vi "Orbit and Timebase Plot (Simulated)_KSS.vi"(8 "error in":errorcluster) -> (0 "error out":errorcluster, 3 "XY Graph":cluster{"probe x":dbl[], "probe y":dbl[]}[](graph))   [LabVIEW 2020]
doc: "This VI demonstrates how to display orbit and timebase plots with a simulated signal.\n\n<B>INSTRUCTIONS</B>:\n1. Specify the <B>sampling info</B>, <B>signal rotating speed</B> and <B>order components</B> contained in the x- and y-axis signals.\n2. For filtered plot, you can specify the <B>orders to display</B> and <B>bandwidth [order]</B>. \n3. Specify the shaft rotating direction, probe orientation and channel pair information in <B> channel properties</B>.\n4. Specify when the display starts and ends to update by setting <B>start [rev]</B> and <B>end [rev]</B> in <B>segment settings</B>.\n5. Specify the <B>timebase buffer size (rev)</B> and <B>orbit buffer size (rev)</B> if you want to view more revolution signals on the plot.\n6. Run the VI.\n\n<B>VIs USED IN THIS EXAMPLE</B>:\n1. OAT Analog Tacho Process.vi\n2. OAT Convert to Even Angle Signal.vi\n3. OAT Order Magnitude and Phase.vi\n4. OAT AC DC Separation.vi\n5. SVX Orbit and Timebase Plot.vi\n6. SVX Combine Filtered and Unfiltered Plots.vi\n7. SVX Buffer Orbit Timebase Plot.vi"
uses:
  <vilib>/addons/_NISVFA/_Shared subVIs/Controls/svc_Channel Info.ctl
  <vilib>/addons/_NISVFA/_Shared subVIs/Controls/svc_Engineering Units Text Ring.ctl
  <vilib>/addons/_NISVFA/_Shared subVIs/Controls/svc_Weighting Filter Text Ring.ctl
  <vilib>/addons/_XControls/Timebase Plot/SVX Timebase.xctl
  <vilib>/addons/_XControls/Orbit Plot/SVX Orbit.xctl
  <vilib>/addons/Sound and Vibration/Order Analysis/Data Presentation/SubVIs/OAT MCM Channel Property.ctl
  <vilib>/addons/_NISVFA/_Shared subVIs/Controls/svc_Window [Dual FFT].ctl
  <vilib>/addons/Sound and Vibration/svt_Calibration/SVL Scale Voltage to EU (N Ch - 1 Info).vi
  <vilib>/addons/Sound and Vibration/svt_Calibration/SVL Scale Voltage to EU (1 Ch).vi
  <vilib>/addons/_NISVFA/_Shared subVIs/Common/svc_Set SV Channel Info.vi
  <vilib>/addons/_NISVFA/_Shared subVIs/Common/svc_Set SV Channel Info (variant).vi
  <vilib>/addons/_NISVFA/_Shared subVIs/Common/SVL Set dB Reference (variant).vi
  <vilib>/addons/_NISVFA/_Shared subVIs/Common/svc_Engineering Units to Unit Label.vi
  <vilib>/addons/_NISVFA/_Shared subVIs/Common/svc_Compute Scale Factor to Convert V to EU.vi
  <vilib>/addons/_NISVFA/_Shared subVIs/Common/svc_Compute Scale Factor to Convert C to EU.vi
  <vilib>/addons/_NISVFA/_Shared subVIs/Common/svc_Set dB ref if Pascal.vi
  <vilib>/addons/_NISVFA/_Shared subVIs/Common/svc_Caller VI Returned in Error Source.vi
  <vilib>/addons/Sound and Vibration/Order Analysis/Tach Process/OAT Analog Tacho Process (1 Tacho).vi
  <vilib>/addons/Sound and Vibration/Order Analysis/Resample Order Tracking/OAT Convert to Even Angle Signal (N Channels).vi
  <vilib>/addons/Sound and Vibration/Order Analysis/Utility/OAT AC DC Separation (N Channels).vi
  <vilib>/addons/Sound and Vibration/Order Analysis/Data Presentation/SVX Orbit and Timebase Plot (Unfiltered).vi
  <vilib>/addons/Sound and Vibration/Order Analysis/Resample Order Tracking/OAT Order Magnitude and Phase (Even Angle Signal, N Channels).vi
  <vilib>/addons/Sound and Vibration/Order Analysis/Data Presentation/SVX Orbit and Timebase Plot (Filtered) (N Ch - M Orders).vi
  <vilib>/addons/Sound and Vibration/Order Analysis/Resample Order Tracking/OAT Full Spectrum (Orbit Plot).vi
  <vilib>/addons/Sound and Vibration/svt_Calibration/SoundVib_Calibration.lvlib
  <vilib>/addons/Sound and Vibration/Order Analysis/Tach Process/SoundVib_TachProcess.lvlib
  <vilib>/addons/Sound and Vibration/Order Analysis/Resample Order Tracking/SoundVib_OrderTracking.lvlib
  <vilib>/addons/Sound and Vibration/Order Analysis/Utility/SoundVib_OAUtility.lvlib
  <vilib>/addons/Sound and Vibration/Order Analysis/Data Presentation/SoundVib_MCMDisplay.lvlib
panel:
  out "orbit/timebase plot out":T1(array[cluster])
  out "subarray":T2(array[cluster])
  in  "channel properties":T3[](array[typedef]) {"probe angle [deg]" max=360; "direction" items=["CCW", "CW"]}
  in  "segment settings":cluster{"start [rev]":dbl, "end [rev]":dbl}={"start [rev]"=0.0, "end [rev]"=inf}
  in  "orbit buffer size (rev)":u32=8
  in  "timebase buffer size (rev)":u32=8
  in  "orders to display":dbl[](array[numeric])=[1.0] format="%.2f"
  in  "y axis order components":T4(array[cluster])=[{"order"=1, "amplitude"=0.5, "phase (deg)"=90.0, "order envelop"=0}, {"order"=2, "amplitude"=1.0, "phase (deg)"=45.0, "order envelop"=2}] {"order envelop" items=["None", "Sine", "Triangle"]}
  in  "channel info":T5={"sensor sensitivity"=1000.0, "engineering units"=1, "dB reference"=1.0, "custom label"="EU", "weighting filter"=0, "pregain"=0.0} {"pregain" format="%.2f"; "weighting filter" items=["Linear", "A-weighting", "B-weighting", "C-weighting", "ITU-R 468-4", "Dolby", "CCITT", "C-message", "Wb", "Wc", "Wd", "We", "Wf", "Wh", "Wj", "Wk", "Wm", "AES17 20 kHz lowpass", "AES17 40 kHz lowpass", "AES17 20 kHz highpass", "AES17 40 kHz highpass"]; "dB reference" format="%^.1e"; "engineering units" items=["custom..."=0, "V"=1, "A"=21, "C"=30, "pC"=31, "s"=32, "-"=29, "Pa"=2, "N"=20, "g"=3, "m/s^2"=4, "m/s"=5, "m"=6, "mm/s"=12, "mm"=13, "micron/s"=14, "micron"=15, "in/s^2"=7, "in/s"=8, "in"=9, "mil/s"=10, "mil"=11, "rad/s^2"=16, "rad/s"=17, "rad"=18, "deg/s^2"=26, "deg/s"=27, "deg"=28, "RPM"=22, "cycle/s^2"=23, "Hz"=24, "cycle"=25, "strain"=19]; "sensor sensitivity" format="%#_5f"}
  in  "x axis order components":T4(array[cluster])=[{"order"=1, "amplitude"=1.0, "phase (deg)"=0.0, "order envelop"=0}, {"order"=2, "amplitude"=0.5, "phase (deg)"=0.0, "order envelop"=2}] {"order envelop" items=["None", "Sine", "Triangle"]}
  in  "sampling info":T8={"sampling frequency"=10000.0, "duration [s]"=10.0} {"sampling frequency" format="%#_6p"}
  in  "signal rotating speed":u16(ring)=3 items=["3000 RPM", "1000-6000 RPM", "6000-1000 RPM", "1000-6000-1000 RPM"]
  in  "bandwidth [order]":dbl=1.0 format="%.2f"
  in  "Tab Control":T9(tab)
  out "Speed profile":cluster{"time [s]":dbl[], "speed [RPM]":dbl[]}(graph)
  out "Vibration signals":waveform(dbl)[](graph)
  out "Timebase Plot":T10(xcontrol)
  out "Orbit Plot":T1(xcontrol)
  out "Full Spectrum":T11(graph)
  # "Simulated Signal Basic Info"
  # "X and Y axes Components\nin Simulated Signal"
  # "Plot Settings"
  # "Filtered Plot Settings"
  # "Channel Settings"
  # "Select Help»Show Context Help and move the cursor over the VI icon for more information."
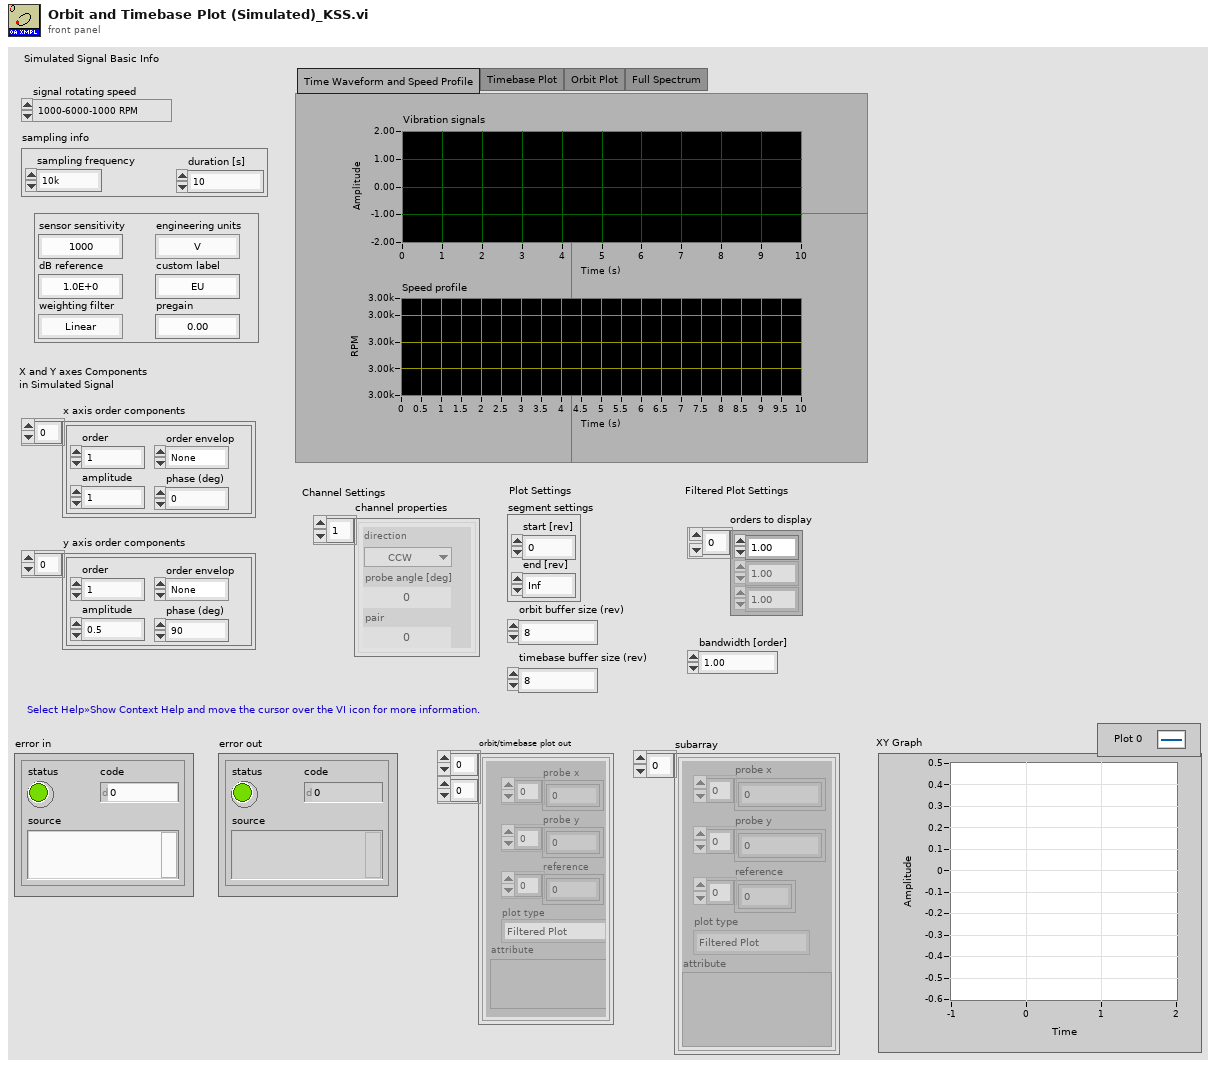
[diagram p1: front panel]
types:
  T1 = cluster{"probe x":dbl[], "probe y":dbl[], "reference":dbl[], "plot type":enum16{"Filtered Plot", "Unfiltered Plot"}, "attribute":variant}[][]
  T2 = cluster{"probe x":dbl[], "probe y":dbl[], "reference":dbl[], "plot type":enum16{"Filtered Plot", "Unfiltered Plot"}, "attribute":variant}[]
  T3 = typedef "OAT MCM Channel Property.ctl" = cluster{"direction":u16, "probe angle [deg]":u16, "pair":u16}
  T4 = cluster{"order":i32, "amplitude":dbl, "phase (deg)":dbl, "order envelop":u16}[]
  T5 = typedef "svc_Channel Info.ctl" = cluster{"sensor sensitivity":dbl, "engineering units":T6, "dB reference":dbl, "custom label":string, "weighting filter":T7, "pregain":dbl}
  T6 = typedef "svc_Engineering Units Text Ring.ctl" = u16
  T7 = typedef "svc_Weighting Filter Text Ring.ctl" = u16
  T8 = cluster{"sampling frequency":dbl, "duration [s]":dbl}
  T9 = enum32{"Time Waveform and Speed Profile", "Timebase Plot", "Orbit Plot", "Full Spectrum"}
  T10 = cluster{"X":dbl[], "Y":dbl[], "reference":dbl[], "plot type":enum16{"Filtered Plot", "Unfiltered Plot"}, "attribute":variant}[][]
  T11 = cluster{"Order 0":dbl, "dOrder":dbl, "magnitude":dbl[]}[]
  T12 = typedef "svc_Window [Dual FFT].ctl" = u32
  T13 = typedef "SoundVib_TachProcess.lvlib/speed profile.ctl" = cluster{"time [s]":dbl[], "speed [RPM]":dbl[]}
  T14 = typedef "svc_Resampled Channel Info.ctl" = cluster{"channel name":string, "description":string, " channel info":T5}
  T15 = typedef "OAT Position Info.ctl" = cluster{"positions [s]":dbl[], "samples/rev":dbl}
  T16 = cluster{"time/rev/rpm":dbl[], "magnitude":dbl[]}[][]
  T17 = typedef "svc_Spectrum Info.ctl" = cluster{"channel name":string, "description":string, "x-axis units":T18, "spectral info":cluster{"spectrum type":T19, "linear/dB":enum16{"linear", "dB"}, "window":u16, "window size":i32, "FFT size":i32}, "engineering units":T6, "custom label":string, "dB reference [EU]":dbl, "peak units":enum16{"rms", "peak", "peak-peak"}, "weighting filter":T7, "spectral density?":bool, "unit label":string, "spectrum skewed?":bool, "complimentary spectrum units":T20}
  T18 = typedef "svc_X-Axis Units.ctl" = u16
  T19 = typedef "svc_Spectrum Type.ctl" = enum16{"FFT Spectrum [complex]", "Amplitude [Magnitude]", "Power [Magnitude^2]", "Cross Spectrum [complex]", "Frequency Response [Complex]"}
  T20 = typedef "svc_Complimentary Spectrum Units.ctl" = enum16{"none", "radians", "degrees", "cycles", "imaginary"}
  T21 = cluster{"forward":cluster{"Order 0":dbl, "dOrder":dbl, "magnitude":dbl[]}, "reverse":cluster{"Order 0":dbl, "dOrder":dbl, "magnitude":dbl[]}}
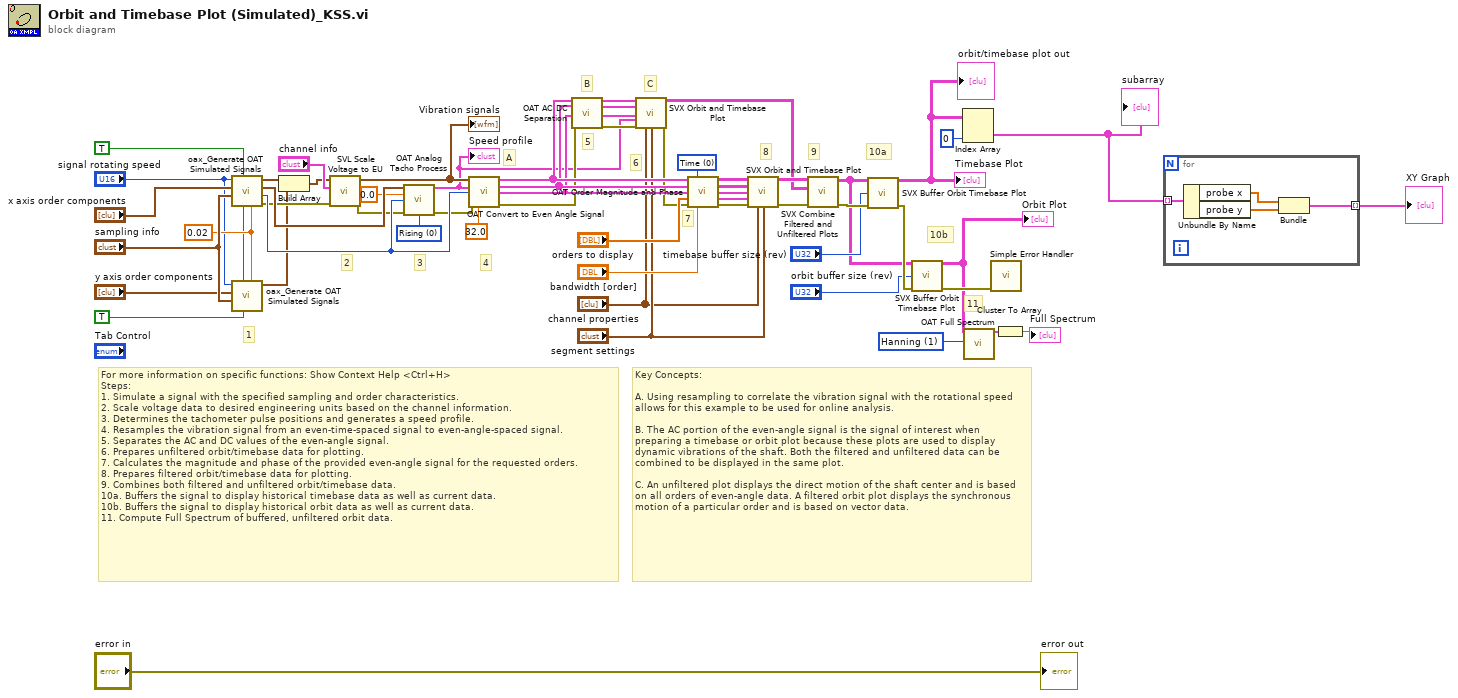
[diagram p0: block diagram]
diagram:
  w9 = T12 1 items=["None"=0, "Hanning"=1, "Hamming"=2, "Blackman-Harris"=3, "Exact Blackman"=4, "Blackman"=5, "Flat Top"=6, "4 Term B-Harris "=7, "7 Term B-Harris"=8, "Low Sidelobe"=9, "Force - Exponential"=10, "Force"=64, "Exponential"=65, "Blackman Nuttall"=11, "Triangle"=30, "Bartlett-Hanning"=31, "Bohman"=32, "Parzen"=33, "Welch"=34, "Kaiser"=60, "Dolph-Chebyshev"=61, "Gaussian"=62] ("window (Hanning)")
  w29 = u16 0 items=["Time", "Revolution", "RPM"] ("X axis selection")
  w39 = u16 0 items=["Rising", "Falling"] ("slope (Rising)")
  w47 = 0.02 ("noise level")
  w46 = TRUE ("add noise?")
  w45 = TRUE ("reset?")
  # "10a"
  # "11"
  # "C"
  # "B"
  # "A"
  # "Key Concepts:\n\nA. Using resampling to correlate the vibration signal with the rotational speed allows for this example to be used for online analysis.\n\nB. The AC portion of the even-angle signal is the signal of interest when preparing a timebase or orbit plot because these plots are used to display dynamic vibrations of the shaft. Both the filtered and unfiltered data can be combined to be displayed in the same plot.\n\nC. An unfiltered plot displays the direct motion of the shaft center and is based on all orders of even-angle data. A filtered orbit plot displays the synchronous motion of a particular order and is based on vector data."
  # "10b"
  # "9"
  # "8"
  # "7"
  # "6"
  # "5"
  # "For more information on specific functions: Show Context Help <Ctrl+H>\nSteps:\n1. Simulate a signal with the specified sampling and order characteristics.\n2. Scale voltage data to desired engineering units based on the channel information.\n3. Determines the tachometer pulse positions and generates a speed profile.\n4. Resamples the vibration signal from an even-time-spaced signal to even-angle-spaced signal.\n5. Separates the AC and DC values of the even-angle signal.\n6. Prepares unfiltered orbit/timebase data for plotting.\n7. Calculates the magnitude and phase of the provided even-angle signal for the requested orders.\n8. Prepares filtered orbit/timebase data for plotting.\n9. Combines both filtered and unfiltered orbit/timebase data.\n10a. Buffers the signal to display historical timebase data as well as current data. \n10b. Buffers the signal to display historical orbit data as well as current data. \n11. Compute Full Spectrum of buffered, unfiltered orbit data."
  # "4"
  # "3"
  # "2"
  # "1"
  n1 = call <vilib>:"oax_Generate OAT Simulated Signals.vi"("noise level"=w47, "add noise?"=w46, "reset?"=w45, "sampling info"="sampling info", "ordercomponents"="x axis order components", "signal rotating speed"="signal rotating speed") -> ("error out"=w51:errorcluster, "pulse/revolution"=w57:i32, "Tach Signal"=w58:waveform(dbl), "Vibration Signal"=w52:waveform(dbl))  [unwired: 2 in]
  n2 = call <vilib>:"oax_Generate OAT Simulated Signals.vi"("noise level"=w47, "add noise?"=w46, "reset?"=w45, "sampling info"="sampling info", "ordercomponents"="y axis order components", "signal rotating speed"="signal rotating speed") -> ("Vibration Signal"=w42:waveform(dbl))  [unwired: 2 in, 3 out]
  n3 = Build Array(w52, w42) -> (w43:waveform(dbl)[])
  n4 = call-poly <vilib>:"SVL Scale Voltage to EU.vi"("error in (no error)"=w51, "channel info"="channel info", "signals [V]"=w43) -> ("error out"=w40:errorcluster, "scaled signals [EU]"=w41:waveform(dbl)[])  [unwired: 6 in, 1 out]
  "Vibration signals" <- w41
  n5 = call-poly <vilib>:"OAT Analog Tacho Process.vi"("analog tacho signal"=w58, "threshold (auto)"=0.0, "pulse/revolution (1)"=w57, "error in (no error)"=w40, "slope (Rising)"=w39) -> ("speed profile"=w21:T13, "error out"=w55:errorcluster)  [unwired: 6 in, 3 out]
  "Speed profile" <- w21
  n6 = call-poly <vilib>:"OAT Convert to Even Angle Signal.vi"("scaled signals [EU]"=w41, "speed profile"=w21, "pulse/revolution (1)"=w57, "error in (no error)"=w55, "max order (auto)"=32.0) -> ("even-angle signals"=w35:cluster{"r0":dbl, "dr":dbl, "Y":dbl[]}[], "even-angle channel info"=w34:T14[], "even-angle position info"=w33:T15, "error out"=w32:errorcluster)  [unwired: 6 in, 1 out]
  n7 = call-poly <vilib>:"OAT AC DC Separation.vi"("even-angle signals"=w35, "even-angle channel info"=w34, "position info"=w33, "error in (no error)"=w32) -> ("even-angle AC signals"=w36:cluster{"r0":dbl, "dr":dbl, "Y":dbl[]}[], "dup even-angle channel info"=w38:T14[], "position info out"=w37:T15, "error out"=w31:errorcluster)  [unwired: 10 in, 2 out]
  n8 = call-poly <vilib>:"SVX Orbit and Timebase Plot.vi"("even-angle signals"=w36, "even-angle channel info"=w38, "even-angle position info"=w37, "speed profile"=w21, "error in (no error)"=w31, "channel properties"="channel properties", "segment settings"="segment settings") -> ("orbit/timebase plot"=w11:T1, "error out"=w22:errorcluster)  [unwired: 5 in, 2 out]
  n9 = call-poly <vilib>:"OAT Order Magnitude and Phase.vi"("even-angle signals"=w35, "x-axis selection"=w29, "even-angle channel info"=w34, "even-angle position info"=w33, "orders to compute (1.0)"="orders to display", "error in (no error)"=w22, "bandwidth [order]"="bandwidth [order]") -> ("magnitudes [RMS]"=w25:T16, "phases [phase lag]"=w24:cluster{"time/rev/rpm":dbl[], "phase":dbl[]}[][], "magnitude/phase position info"=w27:T15, "magnitudes info"=w26:T17[], "error out"=w28:errorcluster)  [unwired: 3 in, 1 out]
  n10 = call-poly <vilib>:"SVX Orbit and Timebase Plot.vi"("magnitudes [RMS]"=w25, "phases [phase lag]"=w24, "magnitude/phase position info"=w27, "magnitudes info"=w26, "error in (no error)"=w28, "channel properties"="channel properties", "segment settings"="segment settings") -> ("orbit/timebase plot"=w12:T1, "error out"=w20:errorcluster)  [unwired: 5 in, 2 out]
  n11 = call <vilib>:"SVX Combine Filtered and Unfiltered Plots.vi"("error in (no error)"=w20, "unfiltered plot"=w11, "filtered plot"=w12) -> ("error out"=w19:errorcluster, "combined plot"=w10:T1)  [unwired: 7 in]
  n12 = call <vilib>:"SVX Buffer Orbit Timebase Plot.vi"("orbit/timebase plot in"=w10, "buffer size (rev)"="timebase buffer size (rev)", "error in (no error)"=w19) -> ("orbit/timebase plot out"=w4:T1, "error out"=w17:errorcluster)  [unwired: 11 in]
  "Timebase Plot" <- w4
  "orbit/timebase plot out" <- w4
  n13 = call <vilib>:"SVX Buffer Orbit Timebase Plot.vi"("orbit/timebase plot in"=w10, "buffer size (rev)"="orbit buffer size (rev)", "error in (no error)"=w17) -> ("orbit/timebase plot out"=w5:T1, "error out"=w15:errorcluster)  [unwired: 11 in]
  "Orbit Plot" <- w5
  n14 = Index Array(array=w4, index (col)=0 ("disabled index (col)")) -> (element=w3:T2)  [unwired: 1 in]
  "subarray" <- w3
  n15 = call-poly <vilib>:"OAT Full Spectrum.vi"("orbit/timebase plot"=w5, "window (Hanning)"=w9) -> ("full spectrum"=w8:T21)  [unwired: 12 in, 5 out]
  n16 = call <vilib>:"Simple Error Handler.vi"("error in (no error)"=w15) -> ()  [unwired: 4 in, 5 out]
  n17 = Cluster To Array(cluster=w8) -> (array=→"Full Spectrum":T11)
  n18 = for {
    tunnel: w3 -> [w62] mode=indexing
    tunnel: [w61] -> w1 mode=indexing
    n19 = Unbundle By Name(w62) -> ("probe x"=w60:dbl[], "probe y"=w59:dbl[])
    n20 = Bundle("probe x"=w60, "probe y"=w59) -> (w61:cluster{"probe x":dbl[], "probe y":dbl[]})  [unwired: 1 in]
  }
  "XY Graph" <- w1
  "error out" <- "error in"
